vi "GetLIDAR.vi"() -> (0 "LIDAR Range (in)":dbl)   [LabVIEW 2019]
uses:
  refnums.vi
  GRNF_DIC.vi
panel:
  in  "offset":dbl
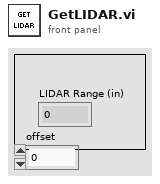
[diagram p1: front panel]
types:
  T1 = typedef "WPI_CounterDevRef.ctl" = cluster{"DevStatus":errorcluster, "CntIndex":T2}
  T2 = typedef "FPGA_CounterCtrSystemIndex.ctl" = enum8{"Ctr 0", "Ctr 1", "Ctr 2", "Ctr 3", "Ctr 4", "Ctr 5", "Ctr 6", "Ctr 7", "Invalid"}
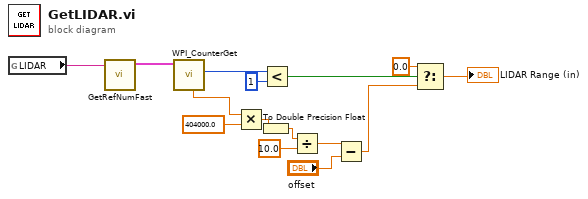
[diagram p0: block diagram]
diagram:
  n1 = global read "refnums.vi" "LIDAR"() -> (w15:string)
  n2 = call-poly "GetRefNumFast.vi"("RefNum Name"=w15) -> ("Device Reference"=w14:T1)  [unwired: 5 in, 1 out]
  n3 = call <vilib>:"WPI_CounterGet.vi"("CounterDevRef in"=w14) -> ("Value"=w10:i32, "Period (sec)"=w2:dbl)  [unwired: 5 in, 4 out]
  n4 = Multiply(x=w2, y=404000.0) -> (x*y=w9:dbl)
  n5 = To Double Precision Float(number=w9) -> (double precision float=w8:dbl)
  n6 = Less?(x=w10, y=1) -> (x < y?=w13:bool)
  n7 = Divide(x=w8, y=10.0) -> (x/y=w6:dbl)
  n8 = Subtract(x=w6, y="offset") -> (x-y=w4:dbl)
  n9 = Select(t=0.0, s=w13, f=w4) -> (s? t:f=→"LIDAR Range (in)":dbl)
